vi "ZeroLoggingSystem.vi"(11 "Error in":errorcluster) -> (0 "Complete":bool=TRUE, 3 "Error out":errorcluster)   [LabVIEW 2024]
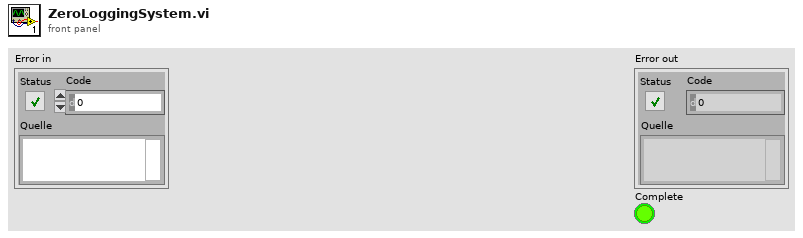
[diagram p1: front panel]
types:
  T1 = cluster{"Devices":refnum<k24>[], "Signals":refnum<k24>[]}
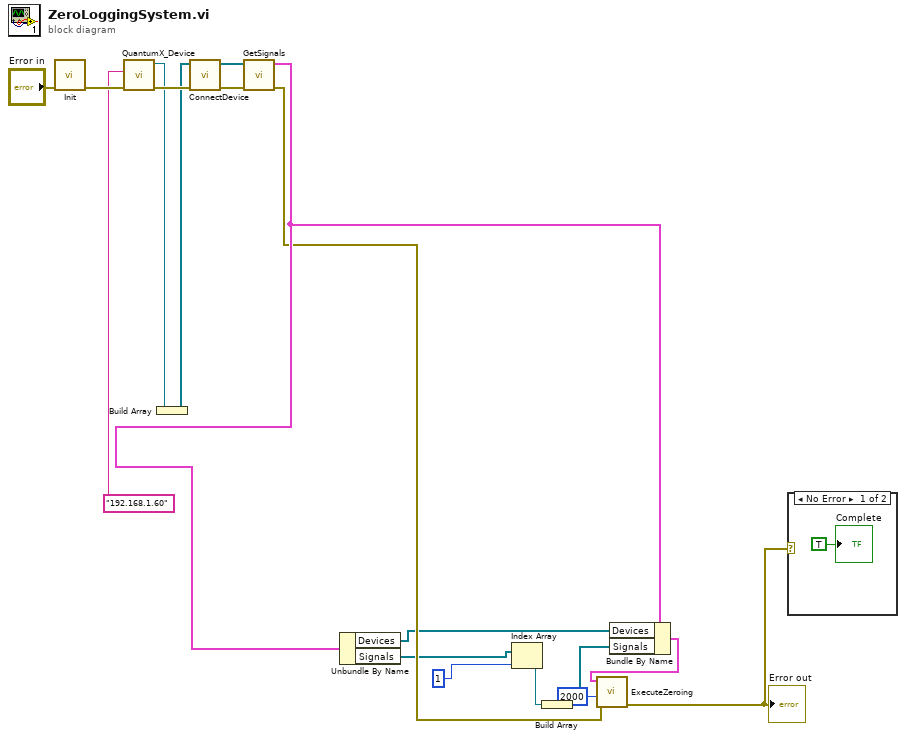
[diagram p0: block diagram]
diagram:
  n1 = call <userlib>:"Init.vi"("Error in"="Error in") -> ("Error out"=w15:errorcluster)  [unwired: 7 in, 2 out]
  n2 = call <userlib>:"QuantumX_Device.vi"("Error in"=w15, "IPAddress"="192.168.1.60" ("IPAddress of QuantumX device")) -> ("Error out"=w16:errorcluster, "Device"=w13:refnum<k24>)  [unwired: 6 in]
  n3 = Build Array(w13) -> (w12:refnum<k24>[])
  n4 = call <userlib>:"ConnectDevice.vi"("Error in"=w16, "Devices"=w12) -> ("Error out"=w18:errorcluster, "Devices"=w17:refnum<k24>[])  [unwired: 7 in, 1 out]
  n5 = call <userlib>:"GetSignals.vi"("Error in"=w18, "Devices"=w17) -> ("Error out"=w10:errorcluster, "DevicesAndSignals"=w11:T1)  [unwired: 8 in]
  n6 = Unbundle By Name(w11) -> ("Devices"=w3:refnum<k24>[], "Signals"=w7:refnum<k24>[])
  n7 = Index Array(array=w7, index=1) -> (element=w8:refnum<k24>)
  n8 = Build Array(w8) -> (w9:refnum<k24>[])
  n9 = Bundle By Name(cluster=w11, "Devices"=w3, "Signals"=w9) -> (w5:T1)
  n10 = call <userlib>:"ExecuteZeroing.vi"("Error in"=w10, "NumberOfMeasurementValuesToUse"=2000, "DevicesAndSignals"=w5) -> ("Error out"=w2:errorcluster)  [unwired: 7 in, 1 out]
  "Error out" <- w2
  n11 = case shown="No Error" w2 {
    frame No Error {
      "Complete" <- TRUE ("Complete")
    }
    frame Error {
    }
  }
